vi "Main - 12-30.vi"() -> ()   [LabVIEW 2013]
uses:
  <vilib>/myRIO/Instrument Drivers/Onboard IO/I2C/typedefs/I2C User Configuration.ctl
  <vilib>/myRIO/Instrument Drivers/Onboard IO/I2C/typedefs/I2C Transfer Rate.ctl
  <vilib>/myRIO/Common/Instrument Driver Framework/myRIO v1.0/DIO/vis/myRIO v1.1 Open DIO.vi
  <vilib>/myRIO/Common/Instrument Driver Framework/myRIO v1.0/I2C/vis/myRIO v1.1 Open I2C.vi
  <vilib>/myRIO/Common/Instrument Driver Framework/myRIO v1.0/UART/vis/myRIO v1.0 Close UART.vi
  <vilib>/myRIO/Common/Instrument Driver Framework/Utilities/vis/Validate Channels.vi
  <vilib>/myRIO/Common/Instrument Driver Framework/myRIO v1.0/DIO/vis/myRIO v1.0 Reserve DIO.vi
  <vilib>/myRIO/Common/Instrument Driver Framework/myRIO v1.0/I2C/vis/myRIO v1.0 Reserve I2C.vi
  <vilib>/myRIO/Common/Instrument Driver Framework/myRIO v1.0/Resource Manager/vis/myRIO v1.0 Reserve Channel List.vi
  <vilib>/myRIO/Common/Instrument Driver Framework/myRIO v1.0/DIO/vis/myRIO v1.0 Build MUX Configuration DIO.vi
  <vilib>/myRIO/Common/Instrument Driver Framework/myRIO v1.0/I2C/vis/myRIO v1.0 Build MUX Configuration I2C.vi
  <vilib>/myRIO/Common/Instrument Driver Framework/myRIO v1.0/Resource Manager/vis/myRIO v1.0 Reserve Channel.vi
  <vilib>/myRIO/Common/Instrument Driver Framework/myRIO v1.0/Resource Manager/vis/myRIO v1.0 Unreserve Channel.vi
  <vilib>/myRIO/Common/Instrument Driver Framework/myRIO v1.0/Resource Manager/vis/myRIO v1.0 Create Configuration List.vi
  <vilib>/myRIO/Common/Instrument Driver Framework/myRIO v1.0/Resource Manager/vis/myRIO v1.0 Build Mutex Name.vi
  <vilib>/myRIO/Common/Instrument Driver Framework/myRIO v1.0/myRIO v1.1 Open.vi
  <vilib>/Utility/VariantDataType/GetNumericInfo.vi
  <vilib>/Utility/error.llb/Error Cluster From Error Code.vi
  <vilib>/myRIO/Common/Instrument Driver Framework/Utilities/vis/IO Manager.vi
  <vilib>/myRIO/Common/Instrument Driver Framework/Utilities/vis/Configuration Manager.vi
  <vilib>/myRIO/Common/Instrument Driver Framework/myRIO v1.0/Resource Manager/vis/myRIO v1.0 Configure IO.vi
  <vilib>/myRIO/Common/Instrument Driver Framework/myRIO v1.0/myRIO v1.0 Close.vi
  <vilib>/myRIO/Common/Instrument Driver Framework/myRIO v1.0/I2C/vis/myRIO v1.0 Configure I2C.vi
  <vilib>/myRIO/Common/Instrument Driver Framework/myRIO v1.0/I2C/vis/myRIO v1.0 Write I2C.vi
  <vilib>/myRIO/Common/Instrument Driver Framework/myRIO v1.0/DIO/vis/myRIO v1.0 Read DIO.vi
  <vilib>/myRIO/Common/Instrument Driver Framework/myRIO v1.0/I2C/vis/myRIO v1.0 Read I2C.vi
  <vilib>/myRIO/Common/Instrument Driver Framework/Utilities/vis/FPGA Ref Manager.vi
  <vilib>/myRIO/Common/Instrument Driver Framework/myRIO v1.0/myRIO v1.0 Reset FPGA.vi
  <vilib>/myRIO/Instrument Drivers/Utilities/Utilities.lvlib
  <vilib>/myRIO/Instrument Drivers/Onboard IO/I2C/I2C.lvlib
  <vilib>/myRIO/Instrument Drivers/Onboard IO/DIO/DIO.lvlib
panel:
  out "INT2":bool
  out "INT1":bool
  out "INT_SOURCE register":bool[](array[boolean])
  out "Waveform Chart":cluster{i16, i16, i16}(graph)
  out "DATAX0 - DATAZ1":u8[](array[numeric]) format="%x"
  out "Z":i16
  out "Y":i16
  out "X":i16
  in  "[ESC]":bool
  # "Accelerometer demo"
  # "D = data ready\n1T = single-tap\n2T = double-tap"
  # "A = activity\nI = inactivity\nF = free fall"
  # "W = watermark\nO = overrun"
  # "D   1T  2T   A    I     F    W   O"
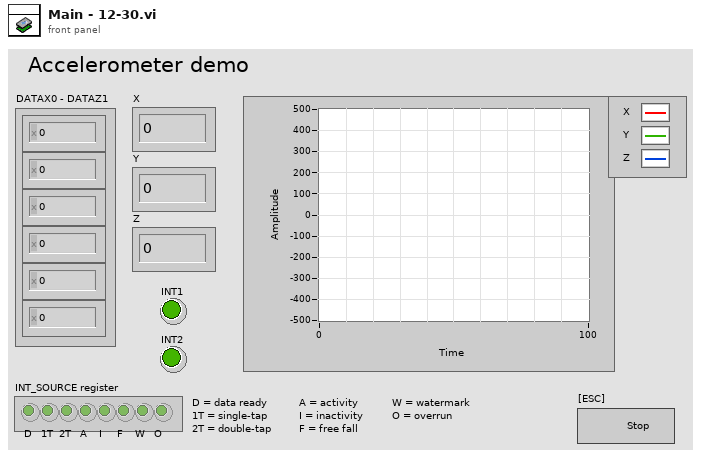
[diagram p1: front panel]
types:
  T1 = typedef "I2C.lvlib/I2C User Configuration.ctl" = cluster{"I2C Transfer Rate":T2}
  T2 = typedef "I2C.lvlib/I2C Transfer Rate.ctl" = enum16{"Standard Mode (100 kbps)", "Fast Mode (400 kbps)"}
  T3 = typedef "I2C.lvlib/I2C Reference.ctl" = cluster{"myRIO Reference":T4, "I2C Channels Enum":T8, "I2C Configuration":T9}
  T4 = typedef "myRIO Generic Hardware Reference.ctl" = cluster{"myRIO Model":T5, "myRIO Hardware Reference":T6}
  T5 = typedef "Hardware Version Enum.ctl" = enum16{"Unknown", "myRIO-1900", "myRIO-1950"}
  T6 = typedef "myRIO v1.0 Reference.ctl" = cluster{"Generic FPGA Reference":T7, "Allow multiple opens":bool}
  T7 = typedef "Generic FPGA Reference.ctl" = refnum<k20>
  T8 = typedef "I2C Channels Enum.ctl" = enum16{"Not Connected", "A/I2C", "B/I2C"}
  T9 = typedef "I2C.lvlib/I2C Configuration.ctl" = cluster{"I2C Transfer Rate":T2}
  T10 = typedef "DIO.lvlib/DIO Reference.ctl" = cluster{"myRIO Reference":T4, "DIO Channels List":T11}
  T11 = typedef "DIO Channels List.ctl" = T12[]
  T12 = typedef "DIO Channels Enum.ctl" = enum16{"Not Connected", "C/DIO0", "C/DIO1", "C/DIO2", "C/DIO3", "C/DIO4", "C/DIO5", "C/DIO6", "C/DIO7", "A/DIO0", "A/DIO1", "A/DIO2", "A/DIO3", "A/DIO4", "A/DIO5", "A/DIO6", "A/DIO7", "A/DIO8", "A/DIO9", "A/DIO10", "A/DIO11", "A/DIO12", "A/DIO13", "A/DIO14", "A/DIO15", "B/DIO0", "B/DIO1", "B/DIO2", "B/DIO3", "B/DIO4", "B/DIO5", "B/DIO6", "B/DIO7", "B/DIO8", "B/DIO9", "B/DIO10", "B/DIO11", "B/DIO12", "B/DIO13", "B/DIO14", "B/DIO15", "LED0", "LED1", "LED2", "LED3", "Button0"}
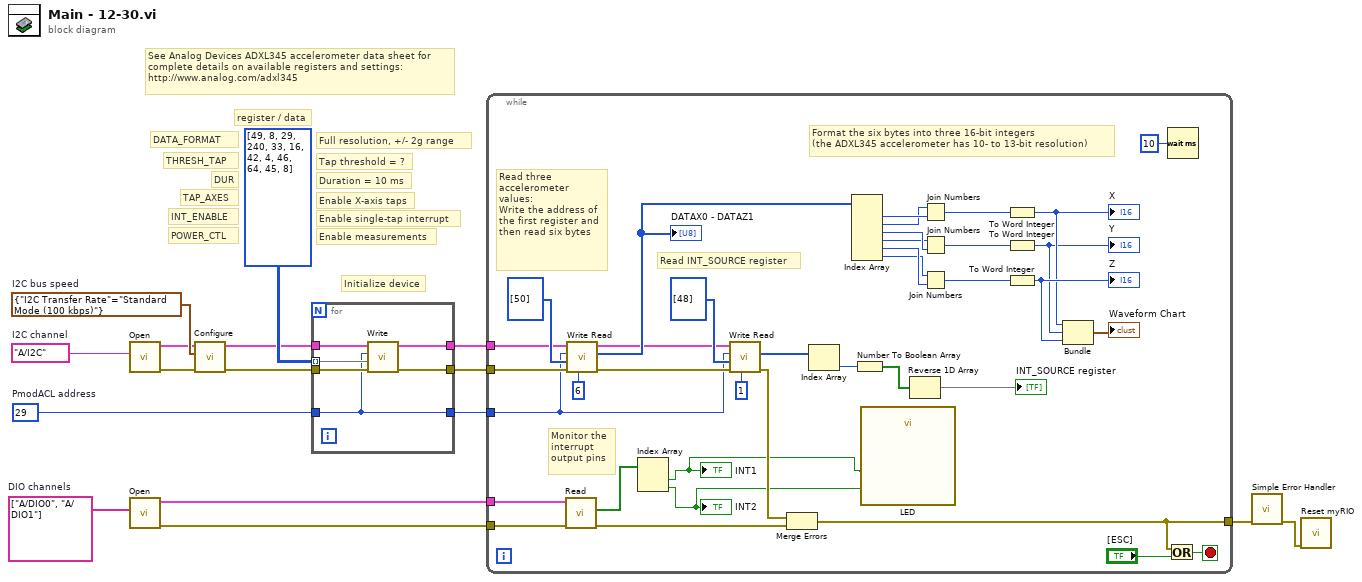
[diagram p0: block diagram]
diagram:
  w1 = tag[] ["A/DIO0", "A/DIO1"]  # DIO channels
  w13 = T1 {"I2C Transfer Rate"=enum."Standard Mode (100 kbps)"}  # I2C bus speed
  w14 = tag "A/I2C"  # I2C channel
  w4 = u8 29  # PmodACL address
  # "Enable X-axis taps"
  # "TAP_AXES"
  # "Initialize device"
  # "Enable measurements"
  # "Enable single-tap interrupt"
  # "Duration = 10 ms"
  # "Tap threshold = ?"
  # "See Analog Devices ADXL345 accelerometer data sheet for\ncomplete details on available registers and settings:\nhttp://www.analog.com/adxl345"
  # "POWER_CTL"
  # "INT_ENABLE"
  # "DUR"
  # "THRESH_TAP"
  # "Full resolution, +/- 2g range"
  # "DATA_FORMAT"
  # "register / data"
  n1 = call <vilib>:"Open.vi"("Channel Name"=w14) -> ("error out"=w11:errorcluster, "I2C Ref Out"=w12:T3)  [unwired: 9 in]
  n2 = call <vilib>:"Open.vi"("Channel Names"=w1) -> ("error out"=w3:errorcluster, "DIO Ref Out"=w2:T10)  [unwired: 9 in]
  n3 = call <vilib>:"Configure.vi"("error in (no error)"=w11, "I2C User Configuration"=w13, "I2C Ref In"=w12) -> ("error out"=w5:errorcluster, "I2C Ref Out"=w6:T3)  [unwired: 7 in]
  n4 = for {
    tunnel: [w22] -> w10
    tunnel: [w21] -> w9
    tunnel: [w17] -> w8
    tunnel: u8[][] [[49, 8], [29, 240], [33, 16], [42, 4], [46, 64], [45, 8]] ("Bytes to Write") -> [w20] mode=indexing
    tunnel: w6 -> [w19]
    tunnel: w5 -> [w18]
    tunnel: w4 -> [w17]
    n5 = call <vilib>:"Write.vi"("error in (no error)"=w18, "Bytes to Write"=w20, "Slave Address (7-bit)"=w17, "I2C Ref In"=w19) -> ("error out"=w22:errorcluster, "I2C Ref Out"=w21:T3)  [unwired: 6 in]
  }
  n6 = while {
    tunnel: [w26] -> w15
    tunnel: w8 -> [w36]
    tunnel: w10 -> [w49]
    tunnel: w9 -> [w48]
    tunnel: w3 -> [w30]
    tunnel: w2 -> [w29]
    stop <- w60 stop-if-true
    # "Monitor the\ninterrupt\noutput pins"
    # "Read INT_SOURCE register"
    # "Read three accelerometer values:\nWrite the address of the first register and then read six bytes"
    # "Format the six bytes into three 16-bit integers\n(the ADXL345 accelerometer has 10- to 13-bit resolution)"
    n7 = call <vilib>:"Read.vi"("error in (no error)"=w30, "DIO Ref In"=w29) -> ("error out"=w27:errorcluster, "Values"=w25:bool[])  [unwired: 7 in, 1 out]
    n8 = call <vilib>:"Write Read.vi"("Byte Count"=u32 6, "error in (no error)"=w49, "Bytes to Write"=u8[] [50], "Slave Address (7-bit)"=w36, "I2C Ref In"=w48) -> ("error out"=w37:errorcluster, "Bytes Read"=w41:u8[], "I2C Ref Out"=w38:T3)  [unwired: 3 in]
    "DATAX0 - DATAZ1" <- w41
    n9 = Index Array "Index Array"(array=w25) -> (element #1=w24:bool, element #2=w23:bool)  [unwired: 2 in]
    "INT1" <- w24
    "INT2" <- w23
    n10 = call <vilib>:"Write Read.vi"("Byte Count"=u32 1, "error in (no error)"=w37, "Bytes to Write"=u8[] [48], "Slave Address (7-bit)"=w36, "I2C Ref In"=w38) -> ("error out"=w28:errorcluster, "Bytes Read"=w35:u8[])  [unwired: 3 in, 1 out]
    n11 = Merge Errors(w28, w27) -> (w26:errorcluster)
    n12 = Index Array "Index Array"(array=w35) -> (element=w34:u8)  [unwired: 1 in]
    n13 = Index Array "Index Array"(array=w41) -> (element #1=w47:u8, element #2=w46:u8, element #3=w45:u8, element #4=w44:u8, element #5=w43:u8, element #6=w42:u8)  [unwired: 6 in]
    n14 = Number To Boolean Array(number=w34) -> (Boolean array=w33:bool[])
    n15 = call "LED"("LED0"=w24, "LED1"=w23) -> ()  [unwired: 25 in, 1 out]
    n16 = Reverse 1D Array(array=w33) -> (reversed array=→"INT_SOURCE register":bool[])
    n17 = Join Numbers(hi=w46, lo=w47) -> ((hi.lo)=w58:u16)
    n18 = Join Numbers(hi=w44, lo=w45) -> ((hi.lo)=w57:u16)
    n19 = Join Numbers(hi=w42, lo=w43) -> ((hi.lo)=w56:u16)
    n20 = To Word Integer(number=w58) -> (16bit integer=w53:i16)
    "X" <- w53
    n21 = To Word Integer(number=w57) -> (16bit integer=w52:i16)
    "Y" <- w52
    n22 = To Word Integer(number=w56) -> (16bit integer=w55:i16)
    "Z" <- w55
    n23 = Bundle "Bundle"(w53, w52, w55) -> (→"Waveform Chart":cluster{i16, i16, i16})  [unwired: 1 in]
    n24 = Or(x=w26, y="[ESC]") -> (x .or. y?=w60:bool)
    n25 = Wait (ms)(milliseconds to wait=u32 10) -> ()  [unwired: 1 out]
  }
  n26 = call <vilib>:"Simple Error Handler.vi"("error in (no error)"=w15) -> ("error out"=w16:errorcluster)  [unwired: 4 in, 4 out]
  n27 = call <vilib>:"Reset myRIO.vi"("error in (no error)"=w16) -> ()  [unwired: 10 in, 1 out]
